vi "S2C_VLFT10_Proc_GetSwVersion.vi"(8 "Error In":errorcluster) -> (0 "Error Out":errorcluster, 2 "Found?":bool, 3 "ItemValue":string)   [LabVIEW 2015]
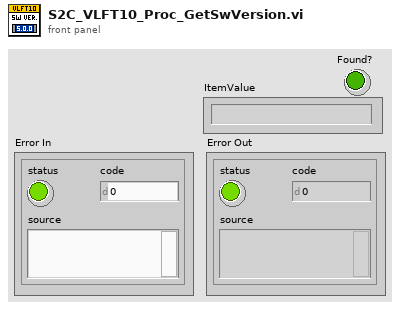
[diagram p1: front panel]
types:
  T1 = cluster{"Detected":cluster{"Items":cluster{"Name":string, "Version":string}[]}}
  T2 = cluster{"Partition":string, "Message":string, "M_ChassisSerialNumber":string, "M_SystemVersion":string, "M_Embodiment":string, "M_LastUpdateDatetime":string, "M_IsConsistent":bool, "M_NeedsConfirmation":bool, "M_ConfigurationData":string}
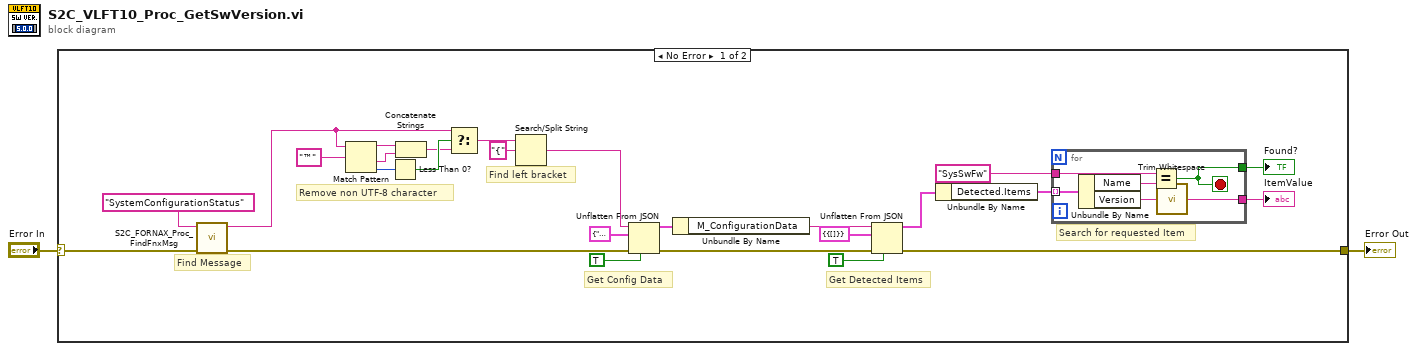
[diagram p0: block diagram]
diagram:
  n1 = case shown="No Error" "Error In" {
    selector: "Error In" -> [w7 w35]
    tunnel: [w11 w35] -> w1
    frame No Error {
      # "Find Message"
      # "Search for requested Item"
      # "Find left bracket"
      # "Remove non UTF-8 character"
      # "Get Detected Items"
      # "Get Config Data"
      n2 = call "S2C_FORNAX_Proc_FindFnxMsg.vi"("Error In"=w7, "MsgName"="SystemConfigurationStatus") -> ("Error Out"=w6:errorcluster, "Message"=w4:string)  [unwired: 8 in]
      n3 = Match Pattern(string=w4, regular expression="™") -> (before substring=w25:string, after substring=w24:string, offset past match=w23:i32)  [unwired: 1 in, 1 out]
      n4 = Less Than 0?(x=w23) -> (x < 0?=w22:bool)
      n5 = Concatenate Strings(w25, w24) -> (w21:string)
      n6 = Select(t=w4, s=w22, f=w21) -> (s? t:f=w15:string)
      n7 = Search/Split String(string=w15, search string/char (-)="{") -> (match + rest of string=w12:string)  [unwired: 1 in, 2 out]
      n8 = Unflatten From JSON(JSON string=w12, type and defaults=T2 {"Partition"="", "Message"="", "M_ChassisSerialNumber"="", "M_SystemVersion"="", "M_Embodiment"="", "M_LastUpdateDatetime"="", "M_IsConsistent"=FALSE, "M_NeedsConfirmation"=FALSE, "M_ConfigurationData"=""}, default null elements? (F)=TRUE, error in (no error)=w6) -> (value=w28:T2, error out=w17:errorcluster)  [unwired: 3 in]
      n9 = Unbundle By Name(w28) -> ("M_ConfigurationData"=w16:string)
      n10 = Unflatten From JSON(JSON string=w16, type and defaults=T1 {"Detected"={"Items"=[]}}, default null elements? (F)=TRUE, error in (no error)=w17) -> (value=w13:T1, error out=w11:errorcluster)  [unwired: 3 in]
      n11 = Unbundle By Name(w13) -> ("Detected.Items"=w14:cluster{"Name":string, "Version":string}[])
      n12 = for {
        tunnel: w14 -> [w34] mode=indexing
        tunnel: "SysSwFw" ("ItemName") -> [w32]
        tunnel: [w29] -> w9
        tunnel: [w31] -> w8
        stop <- w31 stop-if-true
        n13 = Unbundle By Name(w34) -> ("Name"=w33:string, "Version"=w30:string)
        n14 = Equal?(x=w32, y=w33) -> (x = y?=w31:bool)
        n15 = call <vilib>:"Trim Whitespace.vi"("string"=w30) -> ("trimmed string"=w29:string)  [unwired: 1 in]
      }
      "ItemValue" <- w9
      "Found?" <- w8
    }
    frame Error {
    }
  }
  "Error Out" <- w1
